vi "Write Synthesizer Mode.vi"(10 "Synthesizer Mode":enum16{"Normal", "Low Noise"}(ring), 11 "Signal Generator in":refnum<class "Vector Signal Generator.lvclass">) -> (3 "Signal Generator out":refnum<class "Vector Signal Generator.lvclass">)   [LabVIEW 2020, in "Vector Signal Generator.lvclass"]
uses:
  Vector Signal Generator.lvclass
  Vector Signal Generator.lvclass/Vector Signal Generator.ctl
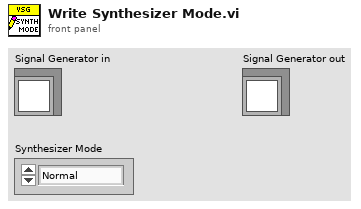
[diagram p1: front panel]
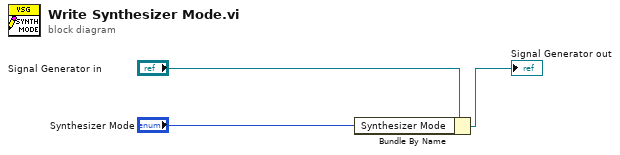
[diagram p0: block diagram]
diagram:
  n1 = Bundle By Name(cluster="Signal Generator in", "Synthesizer Mode"="Synthesizer Mode") -> (→"Signal Generator out":refnum<class "Vector Signal Generator.lvclass">)
